vi "dfd_DFXPSimu Casting (vector)64bits.vi"(5 "quantize output? (T)":bool=TRUE, 7 "op params":T2={"source"=0, "is floating?"=FALSE, "o-mode"=enum."Wrap", "q-mode"=enum."Truncation", "wl"=1, "high limit"=0, "low limit"=0, "iwl"=0, "sign?"=TRUE} {"source" items=["Coef a/k"=0, "Coef b/v"=7, "Input"=1, "Output"=2, "Multiplicand"=3, "Product"=4, "Sum"=5, "Delay"=6, "Gain"=8]}, 8 "filtering statistics in":T6(array[cluster]) {"statistics information"."min value" format="%.2f"; "statistics information"."max value" format="%.2f"; "Quantizer Source" items=["Coefficients a/k"=0, "Coefficients b/v"=7, "Input"=1, "Output"=2, "Multiplicand"=3, "Product"=4, "Sum"=5, "Delay"=6]}, 11 "Value in":T1) -> (0 "filtering statistics out":T6(array[cluster]) {"statistics information"."min value" format="%.2f"; "statistics information"."max value" format="%.2f"; "Quantizer Source" items=["Coefficients a/k"=0, "Coefficients b/v"=7, "Input"=1, "Output"=2, "Multiplicand"=3, "Product"=4, "Sum"=5, "Delay"=6]}, 3 "Value out":T1)   [LabVIEW 2017, in "NI_DigFilter_FXP.lvlib"]
uses:
  <vilib>/addons/Digital Filter Design/NI_DigFilter_FXP.lvlib
  <vilib>/addons/Digital Filter Design/_Objects.llb/dfd_DFXP Data Type (vector).ctl
  <vilib>/addons/Digital Filter Design/_Objects.llb/DFD Quantization Sources.ctl
  <vilib>/addons/Digital Filter Design/_Objects.llb/DFD FXP Statistics Data.ctl
  <vilib>/addons/Digital Filter Design/_Objects.llb/dfd_DFXP Operation Parameter.ctl
  <vilib>/addons/Digital Filter Design/_Objects.llb/dfd_Internal Quantization Srcs.ctl
  <vilib>/addons/Digital Filter Design/NI_DigFilterLicensed.lvlib
panel:
  in  "Value out type":T1
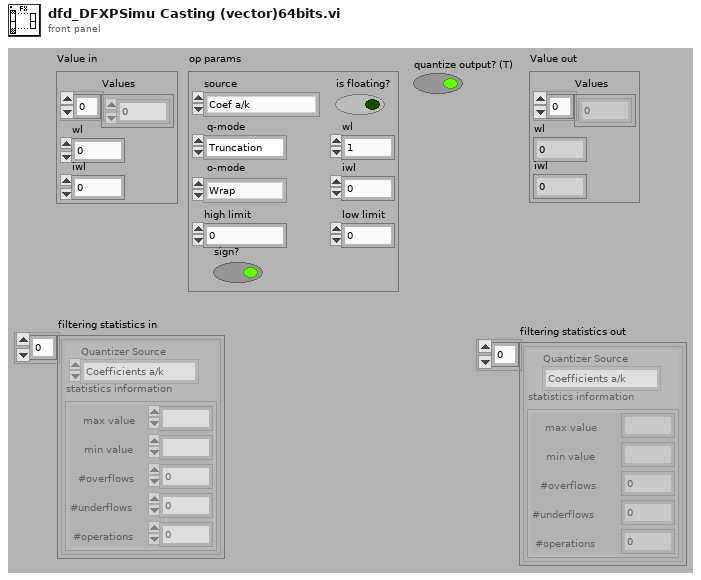
[diagram p1: front panel]
types:
  T1 = typedef "dfd_DFXP Data Type (vector).ctl" = cluster{"Values":i64[], "wl":i16, "iwl":i16}
  T2 = typedef "dfd_DFXP Operation Parameter.ctl" = cluster{"source":T3, "is floating?":bool, "o-mode":enum16{"Saturation", "Wrap"}, "q-mode":enum16{"Nearest", "Truncation"}, "wl":i16, "high limit":i64, "low limit":i64, "iwl":i16, "sign?":bool}
  T3 = typedef "NI_DigFilterLicensed.lvlib/dfd_Internal Quantization Srcs.ctl" = u16
  T4 = typedef "NI_DigFilterLicensed.lvlib/DFD Quantization Sources.ctl" = u16
  T5 = typedef "NI_DigFilterLicensed.lvlib/DFD FXP Statistics Data.ctl" = cluster{"max value":ext, "min value":ext, "#overflows":i32, "#underflows":i32, "#operations":i32}
  T6 = cluster{"Quantizer Source":T4, "statistics information":T5}[]
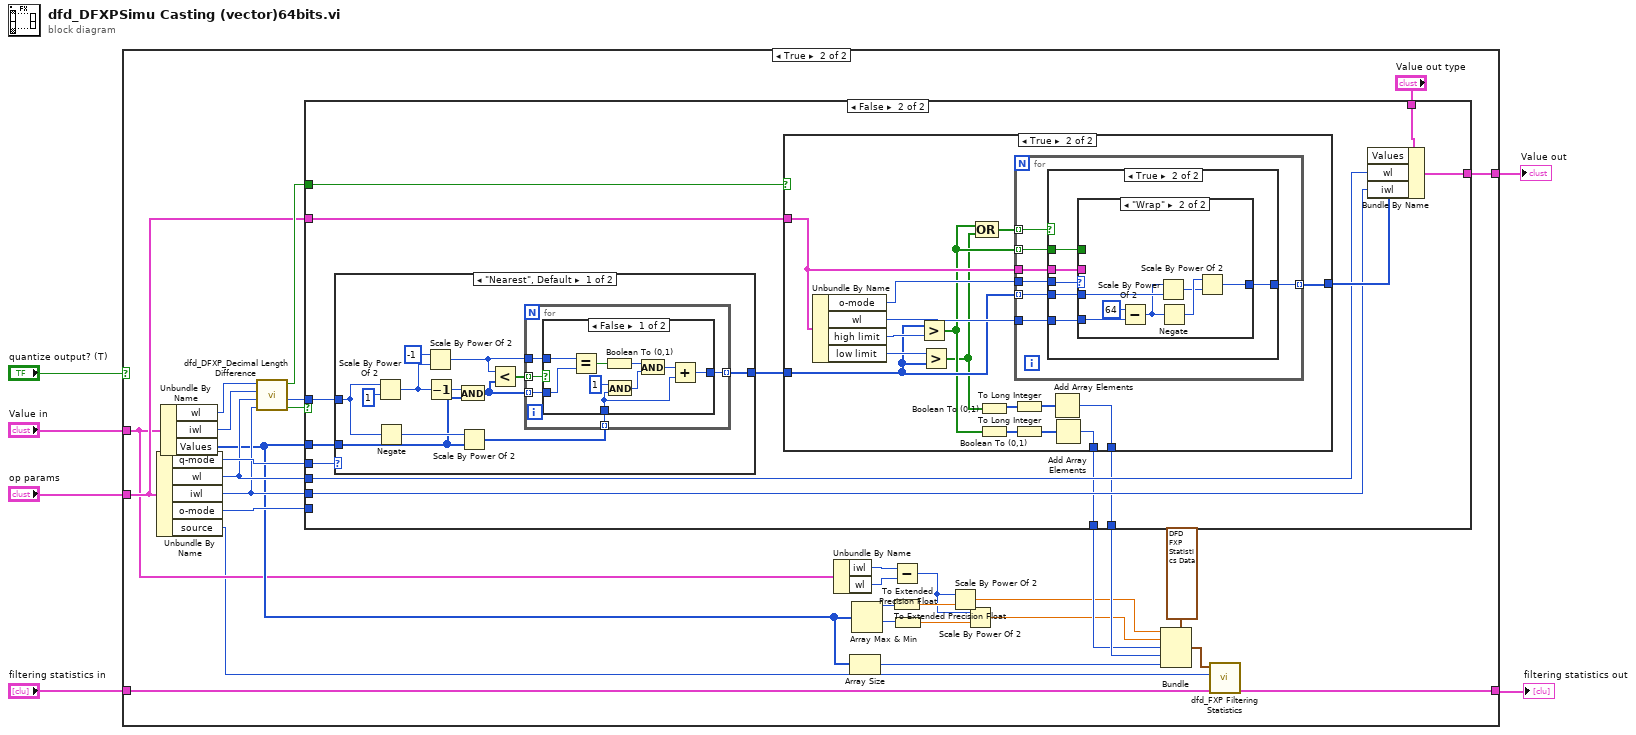
[diagram p0: block diagram]
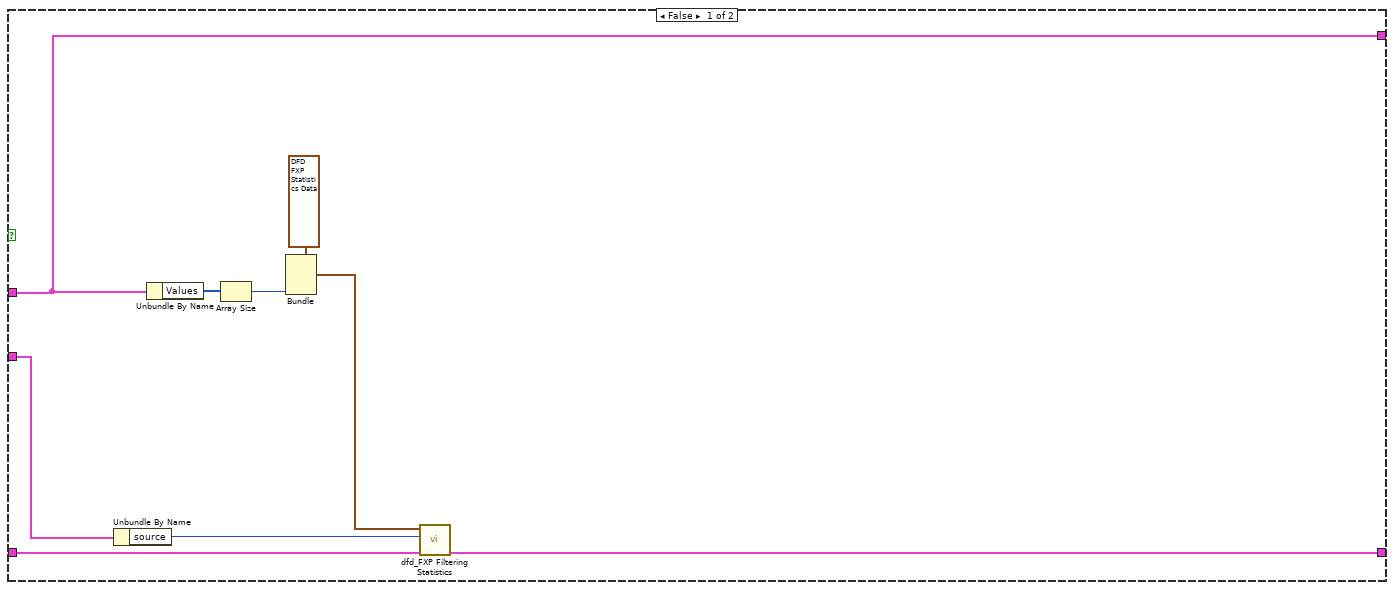
[diagram p2: hidden frame]
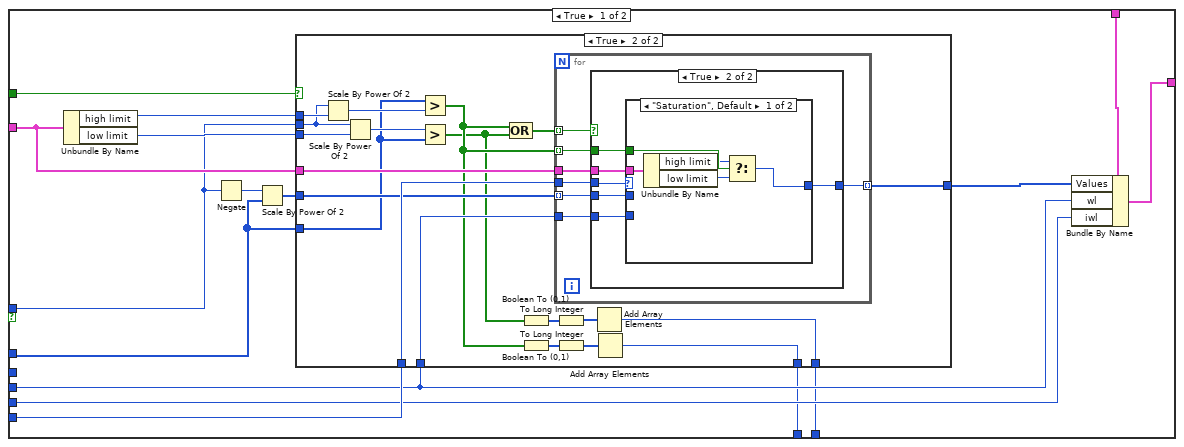
[diagram p3: hidden frame]
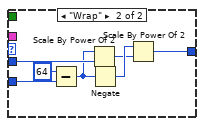
[diagram p6: hidden frame]
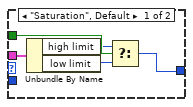
[diagram p9: hidden frame]
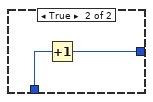
[diagram p10: hidden frame]
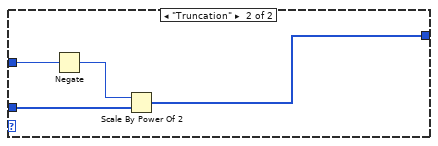
[diagram p11: hidden frame]
diagram:
  n1 = case shown="True" "quantize output? (T)" {
    tunnel: [w14 w35] -> w3
    tunnel: "op params" -> [w15 w38]
    tunnel: "Value in" -> [w14 w33]
    tunnel: "filtering statistics in" -> [w8 w17]
    tunnel: [w7 w16] -> w1
    frame False {
      n2 = Unbundle By Name(w15) -> ("source"=w12:T3)
      n3 = Unbundle By Name(w14) -> ("Values"=w13:i64[])
      n4 = Array Size(array=w13) -> (size(s)=w10:i32)
      n5 = Bundle(cluster=T5 {"max value"=-inf, "min value"=inf, "#overflows"=0, "#underflows"=0, "#operations"=1} ("new data"), "#operations"=w10) -> (w9:T5)  [unwired: 4 in]
      n6 = call <vilib>:"dfd_FXP Filtering Statistics.vi"("filtering statistics in"=w8, "source"=w12, "new data"=w9) -> ("filtering statistics out"=w7:T6)  [unwired: 8 in]
    }
    frame True {
      n7 = Unbundle By Name(w38) -> ("q-mode"=w46:enum16{"Nearest", "Truncation"}, "wl"=w39:i16, "iwl"=w37:i16, "o-mode"=w40:enum16{"Saturation", "Wrap"}, "source"=w32:T3)
      n8 = Unbundle By Name(w33) -> ("wl"=w44:i16, "iwl"=w45:i16, "Values"=w34:i64[])
      n9 = call <vilib>:"dfd_DFXP_Decimal Length Difference.vi"("iwl 2"=w37, "wl 2"=w39, "iwl 1"=w45, "wl 1"=w44) -> ("fwl_diff <= 0?"=w43:bool, "fwl_diff"=w41:i16, "iwl_diff >= 0?"=w42:bool)  [unwired: 5 out]
      n10 = case shown="False" w43 {
        tunnel: w46 -> [_ w122]
        tunnel: w34 -> [w50 w121]
        tunnel: w38 -> [w59 w117]
        tunnel: w42 -> [w51 w119]
        tunnel: w41 -> [w49 w118]
        tunnel: w40 -> [w58 _]
        tunnel: w39 -> [w54 w114]
        tunnel: [w52 w112] -> w35
        tunnel: w37 -> [w53 w113]
        tunnel: "Value out type" -> [w56 w116]
        tunnel: [w48 w111] -> w21
        tunnel: [w47 w110] -> w22
        frame True {
          n11 = Unbundle By Name(w59) -> ("high limit"=w61:i64, "low limit"=w60:i64)
          n12 = Negate(x=w49) -> (-x=w62:i16)
          n13 = Scale By Power Of 2(n=w62, x=w50) -> (x*2^n=w57:i64[])
          n14 = case shown="True" w51 {
            tunnel: w61 -> [_ w83]
            tunnel: w60 -> [_ w82]
            tunnel: w59 -> [_ w78]
            tunnel: w58 -> [_ w77]
            tunnel: w57 -> [w63 w76]
            tunnel: [w63 w75] -> w55
            tunnel: w54 -> [_ w74]
            tunnel: w50 -> [_ w73]
            tunnel: w49 -> [_ w72]
            tunnel: [_ w64] -> w48
            tunnel: [_ w65] -> w47
            frame False {
            }
            frame True {
              n15 = Scale By Power Of 2(n=w72, x=w83) -> (x*2^n=w81:i64)
              n16 = Scale By Power Of 2(n=w72, x=w82) -> (x*2^n=w80:i64)
              n17 = Greater?(x=w73, y=w81) -> (0:w67:bool[])
              n18 = Greater?(x=w80, y=w73) -> (0:w66:bool[])
              n19 = Compound Arithmetic op=OR(w67, w66) -> (w79:bool[])
              n20 = Boolean To (0,1)(Boolean=w66) -> (0, 1=w71:i16[])
              n21 = Boolean To (0,1)(Boolean=w67) -> (0, 1=w70:i16[])
              n22 = for {
                tunnel: w76 -> [w88] mode=indexing
                tunnel: w79 -> [w90] mode=indexing
                tunnel: w67 -> [w89] mode=indexing
                tunnel: w77 -> [w87]
                tunnel: w74 -> [w86]
                tunnel: w78 -> [w85]
                tunnel: [w84] -> w75 mode=indexing
                n23 = case shown="True" w90 {
                  tunnel: w87 -> [_ w97]
                  tunnel: w89 -> [_ w96]
                  tunnel: [w91 w95] -> w84
                  tunnel: w86 -> [_ w94]
                  tunnel: w88 -> [w91 w93]
                  tunnel: w85 -> [_ w92]
                  frame False {
                  }
                  frame True {
                    n24 = case shown="\"Saturation\", Default" w97 {
                      tunnel: w96 -> [w101 _]
                      tunnel: [w98 w108] -> w95
                      tunnel: w94 -> [_ w109]
                      tunnel: w93 -> [_ w107]
                      tunnel: w92 -> [w102 _]
                      frame "Saturation", Default {
                        n25 = Unbundle By Name(w102) -> ("high limit"=w100:i64, "low limit"=w99:i64)
                        n26 = Select(t=w100, s=w101, f=w99) -> (s? t:f=w98:i64)
                      }
                      frame "Wrap" {
                        n27 = Subtract(x=i16 64, y=w109) -> (x-y=w105:i16)
                        n28 = Scale By Power Of 2(n=w105, x=w107) -> (x*2^n=w103:i64)
                        n29 = Negate(x=w105) -> (-x=w104:i16)
                        n30 = Scale By Power Of 2(n=w104, x=w103) -> (x*2^n=w108:i64)
                      }
                    }
                  }
                }
              }
              n31 = To Long Integer(number=w71) -> (32bit integer=w69:i32[])
              n32 = To Long Integer(number=w70) -> (32bit integer=w68:i32[])
              n33 = Add Array Elements(numeric array=w69) -> (sum=w65:i32)
              n34 = Add Array Elements(numeric array=w68) -> (sum=w64:i32)
            }
          }
          n35 = Bundle By Name(cluster=w56, "Values"=w55, "wl"=w54, "iwl"=w53) -> (w52:T1)
        }
        frame False {
          n36 = case shown="\"Nearest\", Default" w122 {
            tunnel: w118 -> [w171 w197]
            tunnel: w121 -> [w174 w194]
            tunnel: [w167 w195] -> w120
            frame "Nearest", Default {
              n37 = Scale By Power Of 2(n=w171, x=i64 1) -> (x*2^n=w172:i64)
              n38 = Negate(x=w171) -> (-x=w177:i16)
              n39 = Scale By Power Of 2(n=-1, x=w172) -> (x*2^n=w170:i64)
              n40 = Decrement(x=w172) -> (x-1=w175:i64)
              n41 = And(x=w175, y=w174) -> (x .and. y?=w169:i64[])
              n42 = Scale By Power Of 2(n=w177, x=w174) -> (x*2^n=w168:i64[])
              n43 = Less?(x=w170, y=w169) -> (x < y?=w166:bool[])
              n44 = for {
                tunnel: w170 -> [w182]
                tunnel: w169 -> [w181] mode=indexing
                tunnel: w168 -> [w180] mode=indexing
                tunnel: [w179] -> w167 mode=indexing
                tunnel: w166 -> [w178] mode=indexing
                n45 = case shown="False" w178 {
                  tunnel: w182 -> [w191 _]
                  tunnel: w181 -> [w190 _]
                  tunnel: w180 -> [w183 w193]
                  tunnel: [w184 w192] -> w179
                  frame False {
                    n46 = Equal?(x=w191, y=w190) -> (x = y?=w188:bool)
                    n47 = Boolean To (0,1)(Boolean=w188) -> (0, 1=w187:i16)
                    n48 = And(x=i64 1, y=w183) -> (x .and. y?=w186:i64)
                    n49 = And(x=w187, y=w186) -> (x .and. y?=w185:i64)
                    n50 = Add(x=w185, y=w183) -> (x+y=w184:i64)
                  }
                  frame True {
                    n51 = Increment(x=w193) -> (x+1=w192:i64)
                  }
                }
              }
            }
            frame "Truncation" {
              n52 = Negate(x=w197) -> (-x=w196:i16)
              n53 = Scale By Power Of 2(n=w196, x=w194) -> (x*2^n=w195:i64[])
            }
          }
          n54 = case shown="True" w119 {
            tunnel: w120 -> [w123 w134]
            tunnel: w117 -> [_ w133]
            tunnel: [w123 w132] -> w115
            tunnel: [_ w125] -> w111
            tunnel: [_ w124] -> w110
            frame False {
            }
            frame True {
              n55 = Unbundle By Name(w133) -> ("o-mode"=w136:enum16{"Saturation", "Wrap"}, "wl"=w135:i16, "high limit"=w139:i64, "low limit"=w138:i64)
              n56 = Greater?(x=w134, y=w139) -> (0:w131:bool[])
              n57 = Greater?(x=w138, y=w134) -> (0:w130:bool[])
              n58 = Compound Arithmetic op=OR(w131, w130) -> (w137:bool[])
              n59 = Boolean To (0,1)(Boolean=w130) -> (0, 1=w129:i16[])
              n60 = Boolean To (0,1)(Boolean=w131) -> (0, 1=w128:i16[])
              n61 = To Long Integer(number=w129) -> (32bit integer=w127:i32[])
              n62 = To Long Integer(number=w128) -> (32bit integer=w126:i32[])
              n63 = for {
                tunnel: w134 -> [w144] mode=indexing
                tunnel: w137 -> [w146] mode=indexing
                tunnel: w131 -> [w145] mode=indexing
                tunnel: w136 -> [w143]
                tunnel: w135 -> [w142]
                tunnel: w133 -> [w141]
                tunnel: [w140] -> w132 mode=indexing
                n64 = case shown="True" w146 {
                  tunnel: w143 -> [_ w153]
                  tunnel: w145 -> [_ w152]
                  tunnel: [w147 w151] -> w140
                  tunnel: w142 -> [_ w150]
                  tunnel: w144 -> [w147 w149]
                  tunnel: w141 -> [_ w148]
                  frame False {
                  }
                  frame True {
                    n65 = case shown="\"Wrap\"" w153 {
                      tunnel: w152 -> [w157 _]
                      tunnel: [w154 w164] -> w151
                      tunnel: w150 -> [_ w165]
                      tunnel: w149 -> [_ w163]
                      tunnel: w148 -> [w158 _]
                      frame "Saturation", Default {
                        n66 = Unbundle By Name(w158) -> ("high limit"=w156:i64, "low limit"=w155:i64)
                        n67 = Select(t=w156, s=w157, f=w155) -> (s? t:f=w154:i64)
                      }
                      frame "Wrap" {
                        n68 = Subtract(x=i16 64, y=w165) -> (x-y=w161:i16)
                        n69 = Scale By Power Of 2(n=w161, x=w163) -> (x*2^n=w159:i64)
                        n70 = Negate(x=w161) -> (-x=w160:i16)
                        n71 = Scale By Power Of 2(n=w160, x=w159) -> (x*2^n=w164:i64)
                      }
                    }
                  }
                }
              }
              n72 = Add Array Elements(numeric array=w127) -> (sum=w124:i32)
              n73 = Add Array Elements(numeric array=w126) -> (sum=w125:i32)
            }
          }
          n74 = Bundle By Name(cluster=w116, "Values"=w115, "wl"=w114, "iwl"=w113) -> (w112:T1)
        }
      }
      n75 = Unbundle By Name(w33) -> ("iwl"=w31:i16, "wl"=w30:i16)
      n76 = Array Size(array=w34) -> (size(s)=w23:i32)
      n77 = Array Max & Min(array=w34) -> (max value=w29:i64, min value=w28:i64)  [unwired: 2 out]
      n78 = Subtract(x=w31, y=w30) -> (x-y=w26:i16)
      n79 = To Extended Precision Float(1:w29) -> (0:w27:ext)
      n80 = To Extended Precision Float(1:w28) -> (0:w25:ext)
      n81 = Scale By Power Of 2(n=w26, x=w27) -> (x*2^n=w20:ext)
      n82 = Scale By Power Of 2(n=w26, x=w25) -> (x*2^n=w19:ext)
      n83 = Bundle(cluster=T5 {"max value"=-inf, "min value"=inf, "#overflows"=0, "#underflows"=0, "#operations"=1} ("new data"), "max value"=w20, "min value"=w19, "#overflows"=w21, "#underflows"=w22, "#operations"=w23) -> (w18:T5)
      n84 = call <vilib>:"dfd_FXP Filtering Statistics.vi"("filtering statistics in"=w17, "source"=w32, "new data"=w18) -> ("filtering statistics out"=w16:T6)  [unwired: 8 in]
    }
  }
  "filtering statistics out" <- w1
  "Value out" <- w3
